vi "templates export template.vi"(7 "Response Header":string, 8 "error out":errorcluster, 10 "First Value":string, 11 "Connection Refnum":T1) -> (0 "error out 2":errorcluster, 1 "empty keyed array":T2, 2 "String":string, 3 "Connection Refnum 2":T1, 5 "HTTP Header":string)   [LabVIEW 2011]
uses:
  Summitek EXT/ODBC/SQL Controls/Connection Refnum.ctl
  ITK EXT/utils/keyedarr.llb/Keyed Array.ctl
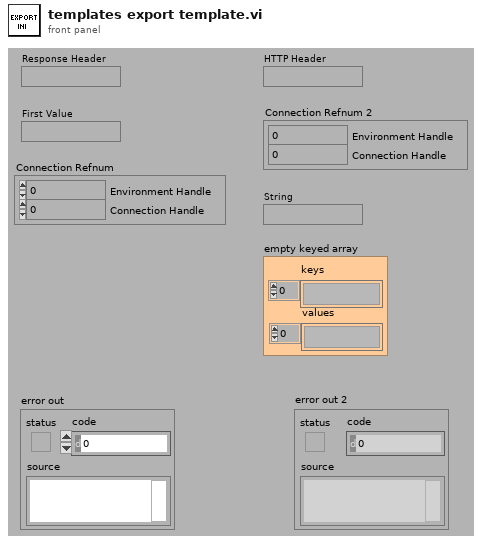
[diagram p1: front panel]
types:
  T1 = typedef "Connection Refnum.ctl" = cluster{"Environment Handle":i32, "Connection Handle":i32}
  T2 = typedef "Keyed Array.ctl" = cluster{"keys":string[], "values":string[]}
  T3 = enum16{"open", "replace", "create", "open or create", "replace or create", "replace or create with confirmation"}
  T4 = typedef "Template Record.ctl" = cluster{"ixTemplate":i32, "sxTemplateId":string, "sDescription":string, "sCreator":string, "tCreationDate":timestamp, "sModifier":string, "tModifiedDate":timestamp, "sType":string, "sStyle":string, "sFormat":string, "dWidth":dbl, "dHeight":dbl, "sFilename":string, "sScript":string, "sLayout":string, "sEditor":string, "sStyleProcess":string}
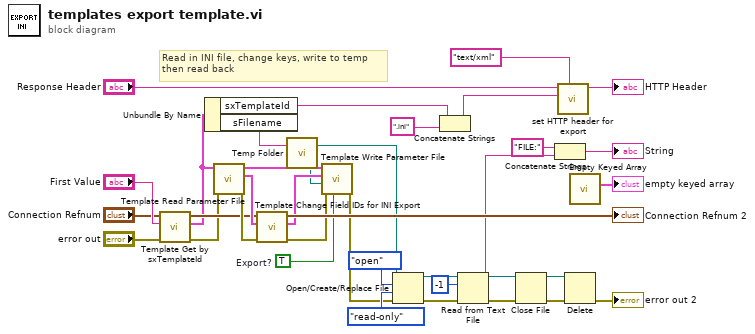
[diagram p0: block diagram]
diagram:
  w33 = TRUE  # Export?
  # "Read in INI file, change keys, write to temp\nthen read back"
  n1 = call "Template Get by sxTemplateId.vi"("error in (no error)"="error out", "sxTemplateId (\"\")"="First Value", "Connection Refnum"="Connection Refnum") -> ("error out"=w22:errorcluster, "Template Record"=w23:T4, "Connection Refnum"=w28:T1)  [unwired: 6 out]
  n2 = Unbundle By Name(w23) -> ("sxTemplateId"=w3:string, "sFilename"=w34:string)
  n3 = call "Template Read Parameter File.vi"("error in (no error)"=w22, "Template Record"=w23) -> ("error out"=w29:errorcluster, "Parameters"=w30:T2, "updated Template Record"=w36:T4)  [unwired: 1 in, 6 out]
  n4 = call "Template Change Field IDs for INI Export.vi"("error in (no error)"=w29, "Parameters"=w30, "Connection Refnum"=w28) -> ("error out"=w32:errorcluster, "Parameters 2"=w31:T2, "Connection Refnum 2"=→"Connection Refnum 2":T1)  [unwired: 6 out]
  n5 = call "Temp Folder.vi"("Relative Path (\"\")"=w34) -> ("Temp Folder"=w10:path)  [unwired: 2 out]
  n6 = call "Template Write Parameter File.vi"("Export?"=w33, "error in (no error)"=w32, "Export Path (\"\")"=w10, "Parameters (empty)"=w31, "Template Record"=w36) -> ("error out"=w9:errorcluster)  [unwired: 1 in, 5 out]
  n7 = Open/Create/Replace File(file path (use dialog)=w10, error in=w9, operation (0:open)=T3."open", access (0:read/write)=enum16{"read/write", "read-only", "write-only"}."read-only") -> (refnum out=w16:refnum<file>, error out=w11:errorcluster)  [unwired: 3 out]
  n8 = Concatenate Strings(w3, ".ini") -> (w2:string)
  n9 = Read from Text File(file (use dialog)=w16, count=-1, error in=w11) -> (refnum out=w13:refnum<file>, text=w8:string, error out=w12:errorcluster)  [unwired: 2 out]
  n10 = Close File(refnum=w13, error in=w12) -> (path=w5:path, error out=w7:errorcluster)
  n11 = Concatenate Strings("FILE:", w8) -> (→"String":string)
  n12 = call "set HTTP header for export.vi"("Content-type (\"application/octet-stream\")"="text/xml" ("Valid Content-Type: (\"text/xml\")"), "filename (\"\")"=w2, "HTTP Header (\"\")"="Response Header") -> ("HTTP Header"=→"HTTP Header":string)  [unwired: 8 out]
  n13 = Delete(path (use dialog)=w5, error in=w7) -> (error out=→"error out 2":errorcluster)  [unwired: 5 out]
  n14 = call "Empty Keyed Array.vi"() -> ("empty keyed array"=→"empty keyed array":T2)  [unwired: 3 out]
